vi "LVRT Serial Init.vi"(6 "stop bits (10: 1 bit)":u16(ring)=10 items=["1 bit"=10, "1.5 bits"=15, "2 bits"=20], 7 "Invert Polarity?":bool=TRUE, 8 "error in (no error)":errorcluster, 9 "parity (0:none)":u16(ring) items=["None", "Odd", "Even", "Mark", "Space"], 10 "data bits (8)":u16=8 min=5 max=8 step=1, 11 "baud rate (9600)":u32=312500) -> (0 "error out":errorcluster, 3 "FPGA Main Reference Out":refnum<k20>)   [LabVIEW 2014]
uses:
  <vilib>/FPGAPlugInAG/myRIO-1900/niLvFpga_Open_myRIO-1900.vi
  <vilib>/FPGAPlugInAG/myRIO-1900/niLvFpga_Reset_myRIO-1900.vi
  <vilib>/FPGAPlugInAG/myRIO-1900/niLvFpga_Run_myRIO-1900.vi
  <vilib>/rvi/interface/nirviOpenFPGA/nirviOpenFPGA.xnode
  FPGA Bitfiles/mySynth_FPGATarget_FPGAMain_WASpsvx+XwM.lvbitx
  FPGA Main.vi
  <vilib>/rvi/interface/nirviMethod/nirviMethod.xnode
  <vilib>/rvi/interface/nirviReadWriteControl/nirviReadWriteControl.xnode
  <vilib>/rvi/errors/niLvFpgaAdjustHostInterfaceError.vi
  <vilib>/rvi/errors/niLvFpgaMergeErrorWithErrorCode.vi
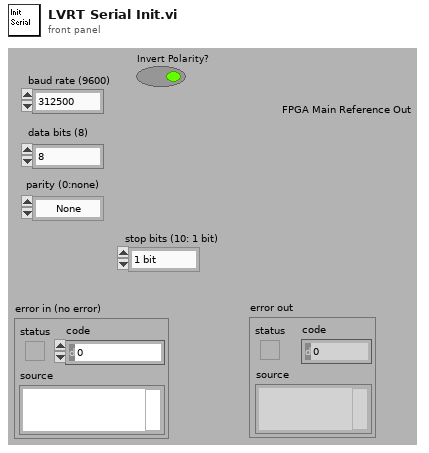
[diagram p1: front panel]
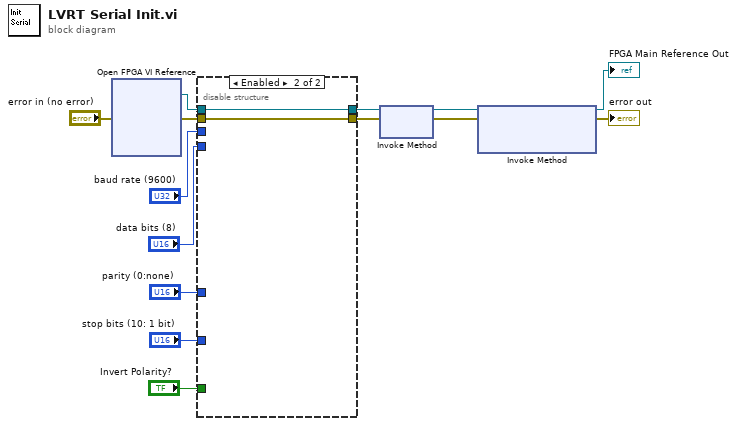
[diagram p0: block diagram]
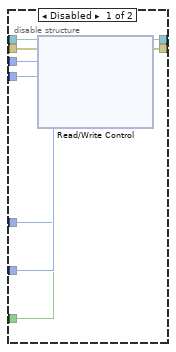
[diagram p2: hidden frame]
diagram:
  n1 = xnode "Open FPGA VI Reference"("error in"="error in (no error)") -> ("FPGA VI Reference Out"=w14:refnum<k20>, "error out"=w13:errorcluster)  [unwired: 1 in]
  n2 = disable-structure shown="Enabled" {
    disable-tunnel: w14 -> [w23 w25]
    disable-tunnel: w13 -> [w22 w24]
    disable-tunnel: "baud rate (9600)" -> [w21 _]
    disable-tunnel: "data bits (8)" -> [w20 _]
    disable-tunnel: "stop bits (10: 1 bit)" -> [w19 _]
    disable-tunnel: "parity (0:none)" -> [w18 _]
    disable-tunnel: "Invert Polarity?" -> [w17 _]
    disable-tunnel: [w16 w24] -> w3
    disable-tunnel: [w15 w25] -> w2
    frame Disabled {
      n3 = xnode "Read/Write Control"("FPGA VI Reference In"=w23, "error in"=w22, "baud rate (9600)"=w21, "data bits (8)"=w20, "parity (0:none)"=w18, "stop bits (10: 1 bit)"=w19, "Invert Polarity?"=w17) -> ("FPGA VI Reference Out"=w15:refnum<k20>, "error out"=w16:errorcluster)
    }
    frame Enabled {
    }
  }
  n4 = xnode "Invoke Method"("FPGA VI Reference In"=w2, "error in"=w3) -> ("FPGA VI Reference Out"=w5:refnum<k20>, "error out"=w4:errorcluster)
  n5 = xnode "Invoke Method"("FPGA VI Reference In"=w5, "error in"=w4) -> ("FPGA VI Reference Out"=→"FPGA Main Reference Out":refnum<k20>, "error out"=→"error out":errorcluster)  [unwired: 1 in]
